vi "DN4_UpDownCounter_GetValue_Ex.vi"(3 "reset updown count?":bool, 4 "error in (no error)":errorcluster, 5 "Task ID":u32) -> (0 "updown count":i32[](array[numeric]), 1 "error out":errorcluster, 2 "Task ID out":u32)   [LabVIEW 2009]
uses:
  Windows/System32/AdvLvDaq.dll
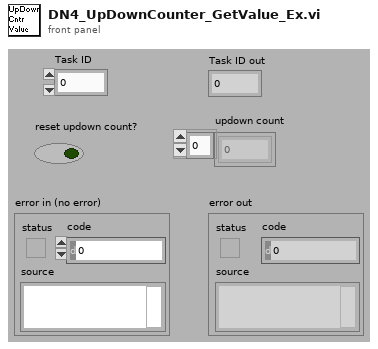
[diagram p1: front panel]
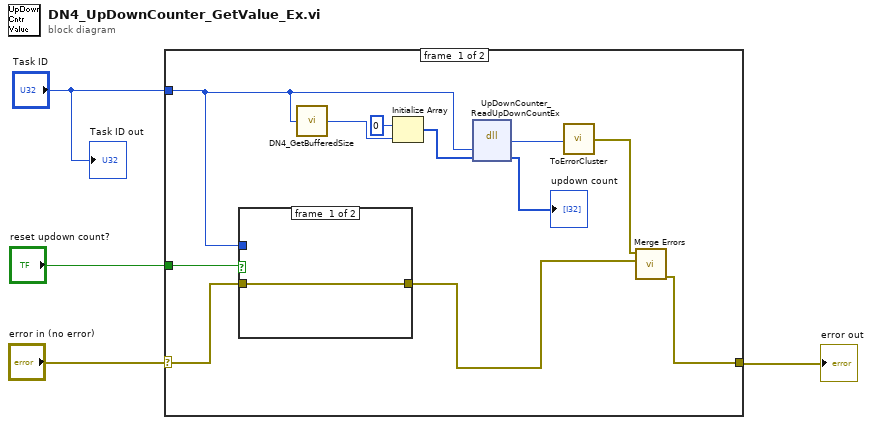
[diagram p0: block diagram]
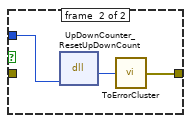
[diagram p2: hidden frame]
diagram:
  n1 = case shown="No Error" "error in (no error)" {
    selector: "error in (no error)" -> [w14 w20]
    tunnel: [w5 w20] -> w3
    tunnel: "Task ID" -> [w10 _]
    tunnel: "reset updown count?" -> [w15 _]
    frame #0 {
      n2 = case shown="True" w15 {
        tunnel: w10 -> [_ w19]
        tunnel: [w16 w17] -> w6
        tunnel: w14 -> [w16 _]
        frame #0 {
        }
        frame #1 {
          n3 = dll-call lib="C:/Windows/System32/AdvLvDaq.dll" fn="UpDownCounter_ResetUpDownCount"("taskID"=w19) -> ("error code"=w18:i32)  [unwired: 4 in, 2 out]
          n4 = call <userlib>:"ToErrorCluster.vi"("error code"=w18) -> ("error out"=w17:errorcluster)
        }
      }
      n5 = call <userlib>:"DN4_GetBufferedSize.vi"("Task ID"=w10) -> ("return type"=w13:i32)
      n6 = Initialize Array(0 ("element"), w13) -> (w11:i32[])
      n7 = dll-call lib="C:/Windows/System32/AdvLvDaq.dll" fn="UpDownCounter_ReadUpDownCountEx"("taskID"=w10, "counts"=w11) -> ("return"=w8:i32, "counts"=→"updown count":i32[])  [unwired: 4 in, 2 out]
      n8 = call <userlib>:"ToErrorCluster.vi"("error code"=w8) -> ("error out"=w7:errorcluster)
      n9 = call <vilib>:"Merge Errors.vi"("error in 2 (no error)"=w6, "error in 1 (no error)"=w7) -> ("error out"=w5:errorcluster)  [unwired: 2 in, 3 out]
    }
    frame #1 {
    }
  }
  "error out" <- w3
  "Task ID out" <- "Task ID"
